vi "SerialTestCreate.vi"(7 "error in (no error)":errorcluster, 8 "Stop Bits":u8(ring)=1 items=["1"=1, "2"=2], 9 "Data Bits":u8(ring)=7 items=["8"=7, "8"=8], 10 "Baudrate":i32(ring)=57600 items=["4800"=4800, "9600"=9600, "19200"=19200, "38400"=38400, "19200"=57600, "115200"=115200], 11 "Port":string(combo)="COM3") -> (3 "Serial Port":u64, 5 "error out":errorcluster)   [LabVIEW 2020]
uses:
  windows/snapmb.dll
panel:
  in  "Parity":string(combo)="E"
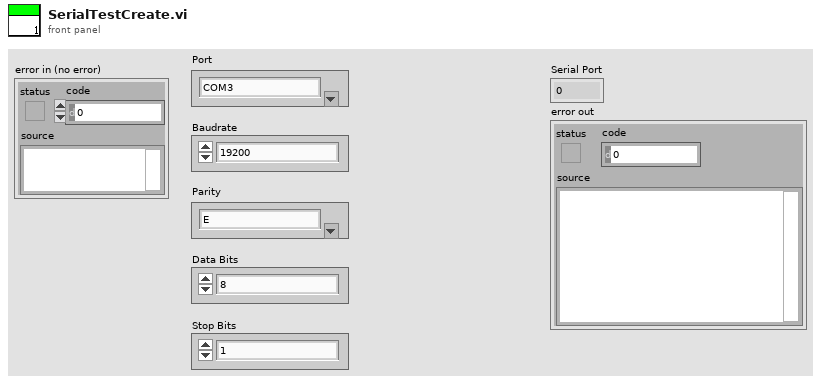
[diagram p1: front panel]
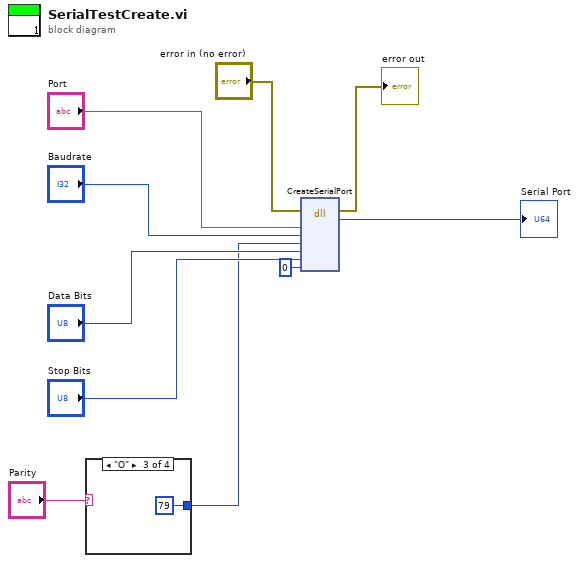
[diagram p0: block diagram]
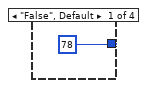
[diagram p2: hidden frame]
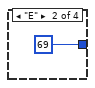
[diagram p3: hidden frame]
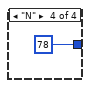
[diagram p4: hidden frame]
diagram:
  n1 = case shown="\"O\"" "Parity" {
    tunnel: [u8 78 u8 69 u8 79 u8 78] -> w1
    frame "False", Default {
    }
    frame "E" {
    }
    frame "O" {
    }
    frame "N" {
    }
  }
  n2 = dll-call lib="D:/SnapMB/LabView/lib/windows/snapmb.dll" fn="CreateSerialPort"(error in="error in (no error)", "Port"="Port", "Baudrate"="Baudrate", "Parity"=w1, "Data Bits"="Data Bits", "Stop Bits"="Stop Bits", "Flow"=u8 0) -> (error out=→"error out":errorcluster, "return type"=→"Serial Port":u64)  [unwired: 8 in, 1 out]
